vi "Drop RPC SubVI in Event Case.vi"(8 "SubDiagram Terminals in":refnum<vi>[](array[refnum]), 9 "gRPC Id EventData Terminal Refnum in":refnum<vi>, 10 "RPC VI in":refnum<vi>, 11 "Subdiagram Refnum in":refnum<vi>) -> ()   [LabVIEW 2019, in "gRPC Template Creation Utility.lvlib"]
uses:
  gRPC Template Creation Utility.lvlib
  <vilib>/Utility/miscctls.llb/LVPointTypeDef.ctl
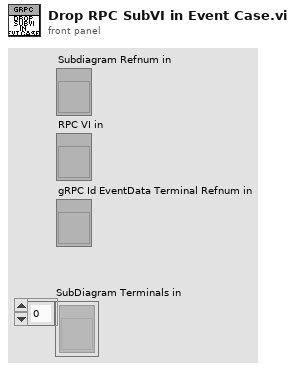
[diagram p1: front panel]
types:
  T1 = typedef "LVPointTypeDef.ctl" = cluster{"Horizontal":i16, "Vertical":i16}
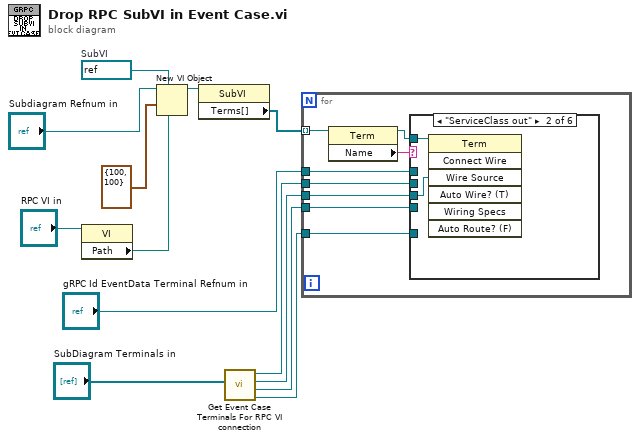
[diagram p0: block diagram]
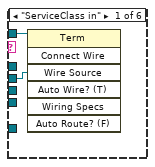
[diagram p2: hidden frame]
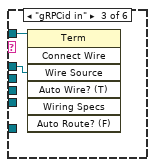
[diagram p3: hidden frame]
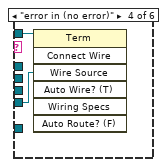
[diagram p4: hidden frame]
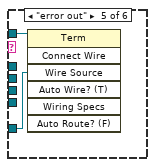
[diagram p5: hidden frame]
diagram:
  w13 = refnum<vi> refnum  # SubVI
  n1 = property class="VI"(reference="RPC VI in") -> ("Path"=w10:path)  [unwired: 1 in, 2 out]
  n2 = New VI Object(vi object class=w13, owner refnum="Subdiagram Refnum in", position/next to=T1 {"Horizontal"=100, "Vertical"=100} ("location"), 6:w10) -> (object refnum=w8:refnum<vi>)  [unwired: 4 in, 1 out]
  n3 = property class="SubVI"(reference=w8) -> ("Terms[]"=w6:refnum<vi>[])  [unwired: 1 in, 2 out]
  n4 = call "Get Event Case Terminals For RPC VI connection.vi"("Event  Inner Case Termianls"="SubDiagram Terminals in") -> ("error out Term"=w2:refnum<vi>, "error in Term"=w3:refnum<vi>, "Service out Term"=w4:refnum<vi>, "Service in Term"=w5:refnum<vi>)  [unwired: 7 in]
  n5 = for {
    tunnel: w6 -> [w21] mode=indexing
    tunnel: "gRPC Id EventData Terminal Refnum in" -> [w18]
    tunnel: w5 -> [w17]
    tunnel: w4 -> [w16]
    tunnel: w3 -> [w15]
    tunnel: w2 -> [w14]
    n6 = property class="Term"(reference=w21) -> (reference out=w19:refnum<vi>, "Name"=w20:string)  [unwired: 1 in, 1 out]
    n7 = case shown="\"ServiceClass out\"" w20 {
      tunnel: w19 -> [w23 w25 w26 w29 w31 _]
      tunnel: w18 -> [_ _ w27 _ _ _]
      tunnel: w17 -> [w22 _ _ _ _ _]
      tunnel: w16 -> [_ w24 _ _ _ _]
      tunnel: w15 -> [_ _ _ w28 _ _]
      tunnel: w14 -> [_ _ _ _ w30 _]
      frame "ServiceClass in" {
        n8 = invoke class="Term" method="Connect Wire"(reference=w23, "Wire Source"=w22) -> ()  [unwired: 5 in, 7 out]
      }
      frame "ServiceClass out" {
        n9 = invoke class="Term" method="Connect Wire"(reference=w25, "Wire Source"=w24) -> ()  [unwired: 5 in, 7 out]
      }
      frame "gRPCid in" {
        n10 = invoke class="Term" method="Connect Wire"(reference=w26, "Wire Source"=w27) -> ()  [unwired: 5 in, 7 out]
      }
      frame "error in (no error)" {
        n11 = invoke class="Term" method="Connect Wire"(reference=w29, "Wire Source"=w28) -> ()  [unwired: 5 in, 7 out]
      }
      frame "error out" {
        n12 = invoke class="Term" method="Connect Wire"(reference=w31, "Wire Source"=w30) -> ()  [unwired: 5 in, 7 out]
      }
      frame Default {
      }
    }
  }
